vi "Update AllChnlParametersHW.vi"(8 "error in (no error)":errorcluster, 11 "BME_DG_System in":refnum<class "BME_DG_System.lvclass">) -> (0 "error out":errorcluster, 3 "BME_DG_System out":refnum<class "BME_DG_System.lvclass">)   [LabVIEW 2009, in "POLARIS BME DG.lvlib" / "BME_DG_System.lvclass"]
doc: "VI updates delays of all channels in hardware.\nIf some SG08p02 cards are in system, SyncLoadAllCards will be called.\n\nLast update 26.11.2012, SyncLoadAllCards added\n\nauthor: Alexander Kessler, Helmholtz-Institut-Jena \nmaintainer: Alexander Kessler: alexander.kessler@uni-jena.de\n\nLast Change: 2012-07-03\n\n\nLicense Agreement for this software:\n\nCopyright (C)\nHelmholtz-Institut-Jena\nFröbelsteg 3\n07743 Jena\nGermany\n\nContact: alexander.kessler@uni-jena.de\n\nThis program is free software; you can redistribute it and/or modify it under the terms of the GNU General Public License as published by the Free Software Foundation; either version 2 of the license, or (at your option) any later version.\n\nThis program is distributed in the hope that it will be useful, but WITHOUT ANY WARRANTY; without even the implied warranty of MERCHANTABILITY or FITNESS FOR A PARTICULAR PURPOSE. See the GNU General License for more details (http://www.gnu.org)."
uses:
  BME_DG_System.lvclass
  BME_DG_System.lvclass/BME_DG_System.ctl
  BME_DG_Base/BME_DG_Base.lvclass
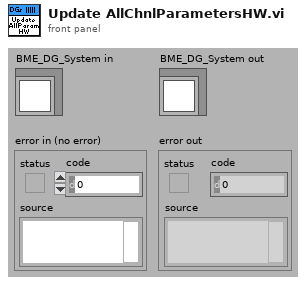
[diagram p1: front panel]
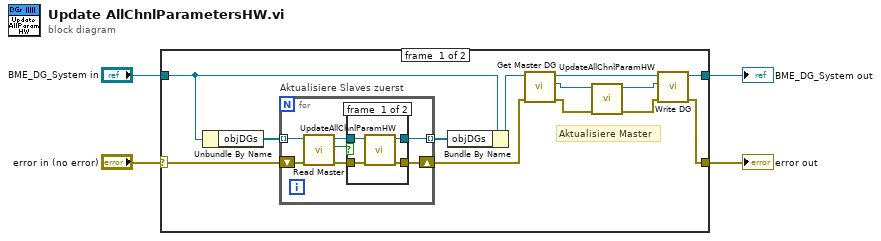
[diagram p0: block diagram]
diagram:
  n1 = case shown="No Error" "error in (no error)" {
    selector: "error in (no error)" -> [w15 w32]
    tunnel: [w5 w32] -> w3
    tunnel: [w10 w31] -> w1
    tunnel: "BME_DG_System in" -> [w17 w31]
    frame #0 {
      # "Aktualisiere Master"
      n2 = Unbundle By Name(w17) -> ("objDGs"=w16:refnum<class "BME_DG_Base.lvclass">[])
      n3 = for "Aktualisiere Slaves zuerst" {
        tunnel: w16 -> [w20] mode=indexing
        tunnel: [w24] -> w14 mode=indexing
        shift-right: [w23] -> w9
        shift-left: w15 -> [w22]
        n4 = call-dynamic "Read Master.vi"("error in (no error)"=w22, "BME_DG_Base in"=w20) -> ("error out"=w21:errorcluster, "Master?"=w19:bool, "BME_DG_Base out"=w18:refnum<class "BME_DG_Base.lvclass">)  [unwired: 6 in, 1 out]
        n5 = case shown="False" w19 {
          tunnel: [w28 w30] -> w24
          tunnel: [w27 w29] -> w23
          tunnel: w21 -> [w26 w29]
          tunnel: w18 -> [w25 w30]
          frame #0 {
            n6 = call-dynamic "UpdateAllChnlParamHW.vi"("error in (no error)"=w26, "BME_DG_Base in"=w25) -> ("error out"=w27:errorcluster, "BME_DG_Base out"=w28:refnum<class "BME_DG_Base.lvclass">)  [unwired: 8 in]
          }
          frame #1 {
          }
        }
      }
      n7 = Bundle By Name(cluster=w17, "objDGs"=w14) -> (w13:refnum<class "BME_DG_System.lvclass">)
      n8 = call "Get Master DG.vi"("error in (no error)"=w9, "BME_DG_System in"=w13) -> ("error out"=w12:errorcluster, "BME_DG_Base.lvclass"=w8:refnum<class "BME_DG_Base.lvclass">, "BME_DG_System out"=w11:refnum<class "BME_DG_System.lvclass">)  [unwired: 7 in]
      n9 = call-dynamic "UpdateAllChnlParamHW.vi"("error in (no error)"=w12, "BME_DG_Base in"=w8) -> ("error out"=w6:errorcluster, "BME_DG_Base out"=w7:refnum<class "BME_DG_Base.lvclass">)  [unwired: 8 in]
      n10 = call "Write DG.vi"("error in (no error)"=w6, "BME_DG_Base"=w7, "BME_DG_System in"=w11) -> ("error out"=w5:errorcluster, "BME_DG_System out"=w10:refnum<class "BME_DG_System.lvclass">)  [unwired: 7 in]
    }
    frame #1 {
    }
  }
  "error out" <- w3
  "BME_DG_System out" <- w1
